vi "Dialog_Enter Loop Iterations.vi"(8 "Error In":errorcluster) -> (0 "Error Out":errorcluster, 2 "Cancelled?":bool, 3 "Macro Commands":T1)   [LabVIEW 2012]
doc: "This VI has no controls.\nThis is a dummy whihc runs when user selects a macro command which does not require any arguments"
uses:
  Custom Controls and Typedefs/Macro_CommandStruct.ctl
  Custom Controls and Typedefs/Macro_Action_List.ctl
  Custom Controls and Typedefs/Macro_ArgumentStruct.ctl
panel:
  in  "Cancel Button":bool
  in  "OK Button":bool
  in  "Iter.No":dbl
  # "Enter the number of iterations for the LOOP"
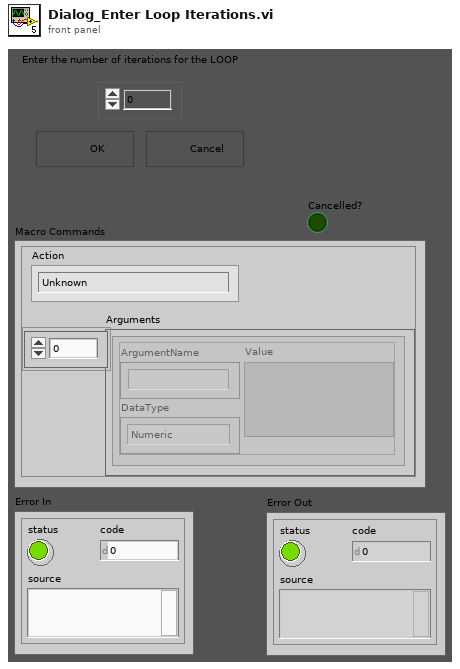
[diagram p1: front panel]
types:
  T1 = typedef "Macro_CommandStruct.ctl" = cluster{"Action":T2, "Arguments":T3[]}
  T2 = typedef "Macro_Action_List.ctl" = enum16{"Unknown", "2D.Frame.Scan", "2D.Line.Scan", "Load.Settings.File", "Move.To.Position", "Pause", "Z.Stack", "LOOP.Start", "LOOP.End"}
  T3 = typedef "Macro_ArgumentStruct.ctl" = cluster{"ArgumentName":string, "DataType":enum16{"Numeric", "String"}, "Value":variant}
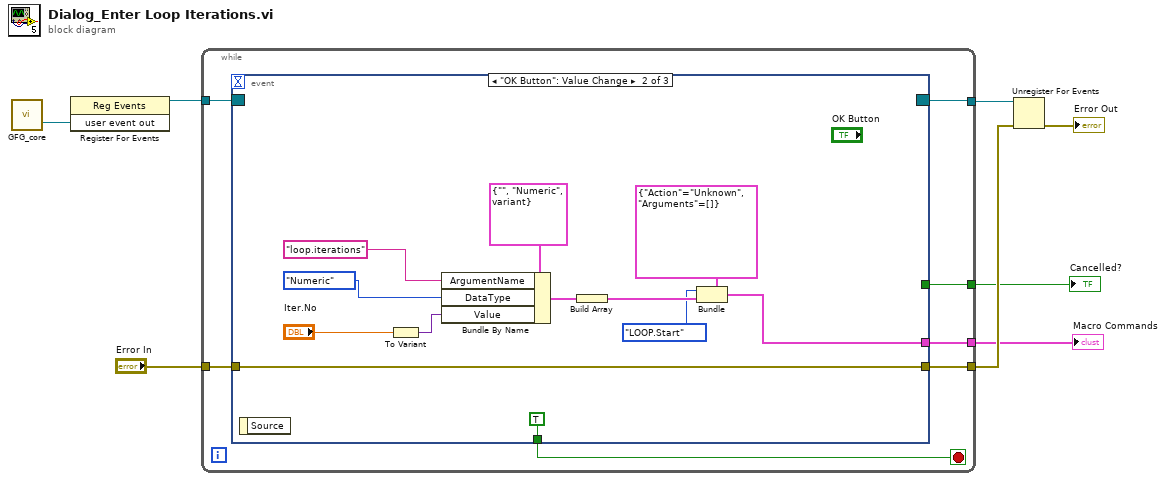
[diagram p0: block diagram]
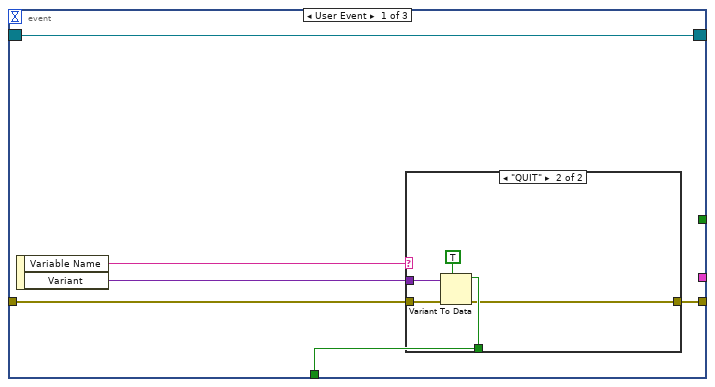
[diagram p2: hidden frame]
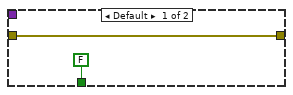
[diagram p3: hidden frame]
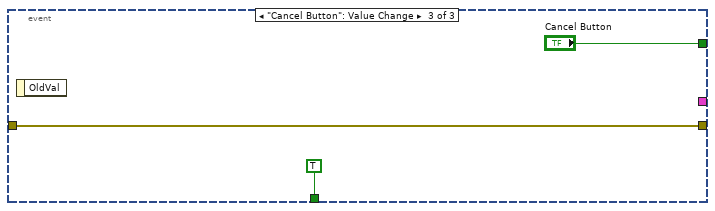
[diagram p4: hidden frame]
diagram:
  n1 = call "GFG_core.vi"() -> ("user event out"=w8:refnum<user-event>)  [unwired: 13 in, 6 out]
  n2 = register-events(w8) -> (reference out=w7:refnum<event-registration>)  [unwired: 2 in, 1 out]
  n3 = while {
    tunnel: w7 -> [w15]
    tunnel: [w14] -> w6
    tunnel: "Error In" -> [w12]
    tunnel: [w11] -> w4
    tunnel: [w10] -> w2
    tunnel: [w9] -> w1
    stop <- w13 stop-if-true
    n4 = event shown="[1] \"OK Button\": Value Change" {
      selector: w15 -> [w21 _ _]
      dyn-events: [w21 _ _] -> w14
      timeout: _ -> [_ _ _]
      tunnel: [w18 TRUE TRUE] -> w13
      tunnel: w12 -> [w17 w30 w42]
      tunnel: [w16 w30 w42] -> w11
      tunnel: [_ w31 _] -> w10
      tunnel: [_ _ "Cancel Button"] -> w9
      event User Event {
        n5 = event-data() -> ("Variable Name"=w20:string, "Variant"=w19:variant)  [unwired: 1 in]
        n6 = case shown="\"QUIT\"" w20 {
          tunnel: w19 -> [_ w27]
          tunnel: [FALSE w26] -> w18
          tunnel: w17 -> [w22 w25]
          tunnel: [w22 w24] -> w16
          frame Default {
          }
          frame "QUIT" {
            n7 = Variant To Data(error in=w25, type=TRUE, Variant=w27) -> (data=w26:bool, error out=w24:errorcluster)
          }
        }
      }
      event "OK Button": Value Change {
        n8 = event-data() -> ()  [unwired: 1 in, 1 out]
        n9 = To Variant(anything="Iter.No") -> (Variant=w37:variant)
        n10 = Bundle By Name(cluster=T3 {"ArgumentName"="", "DataType"=enum."Numeric", "Value"=variant} ("Arguments"), "ArgumentName"="loop.iterations", "DataType"=enum16{"Numeric", "String"}."Numeric", "Value"=w37) -> (w34:T3)
        n11 = Build Array(w34) -> (w33:T3[])
        n12 = Bundle(cluster=T1 {"Action"=enum."Unknown", "Arguments"=[]} ("Macro Commands"), "Action"=Macro_Action_List."LOOP.Start", "Arguments"=w33) -> (w31:T1)
      }
      event "Cancel Button": Value Change {
        n13 = event-data() -> ()  [unwired: 1 in, 1 out]
      }
    }
  }
  "Macro Commands" <- w2
  "Cancelled?" <- w1
  n14 = Unregister For Events(event registration refnum=w6, error in=w4) -> (error out=→"Error Out":errorcluster)
